vi "Init Coil Calibration.vi"(0 "Magnet ID":string, 1 "# Power Supplies":u32(slide)=4 min=1 max=4 step=1 scale=1.0..4.0, 3 "error in (no error)":errorcluster) -> (4 "File Name":string, 5 "I Scale Max":dbl, 6 "Magnet Configuration Data":T1 {"Scale Factors" format="%.3f"; "Offsets" format="%.3f"; "Temp Coef" format="%.4g"; "Maximum Coil Currents" format="%.2g"; "Coil Inductances" format="%.3g"; "Pressure Range" format="%.2f"}, 7 "P Scale Max":dbl, 8 "P Scale Min":dbl, 9 "error out":errorcluster)   [LabVIEW 2018]
doc: "Reads configuration file for the selected magnet from the folder \"Magnet Calibrations\" on the system disk. All comments (lines starting with a '#') are stripped out and the configuration parameters are parsed and output.\nScott Hannahs, NHMFL-FSU, April 1995\nAuthor: Scott Hannahs <sth@magnet.fsu.edu>\nCopyright 2018 Florida State University, All rights reserved."
uses:
  PS Control/Sub Controls/RMPS Magnet Config.ctl
  RMPS Globals.vi
panel:
  # "Tin"
  # "Tout"
  # "Pin"
  # "Pout"
  # "I"
  # "WDTin"
  # "PSEnb"
  # "CellFLT"
  # "WDTout"
  # "BTFlt"
  # "BTvolt"
  # "Va"
  # "Vb"
  # "Vc"
  # "Vd"
  # "Tin"
  # "Tout"
  # "Pin"
  # "Pout"
  # "I"
  # "WDTin"
  # "PSEnb"
  # "CellFLT"
  # "WDTout"
  # "BTFlt"
  # "BTvolt"
  # "Va"
  # "Vb"
  # "Vc"
  # "Vd"
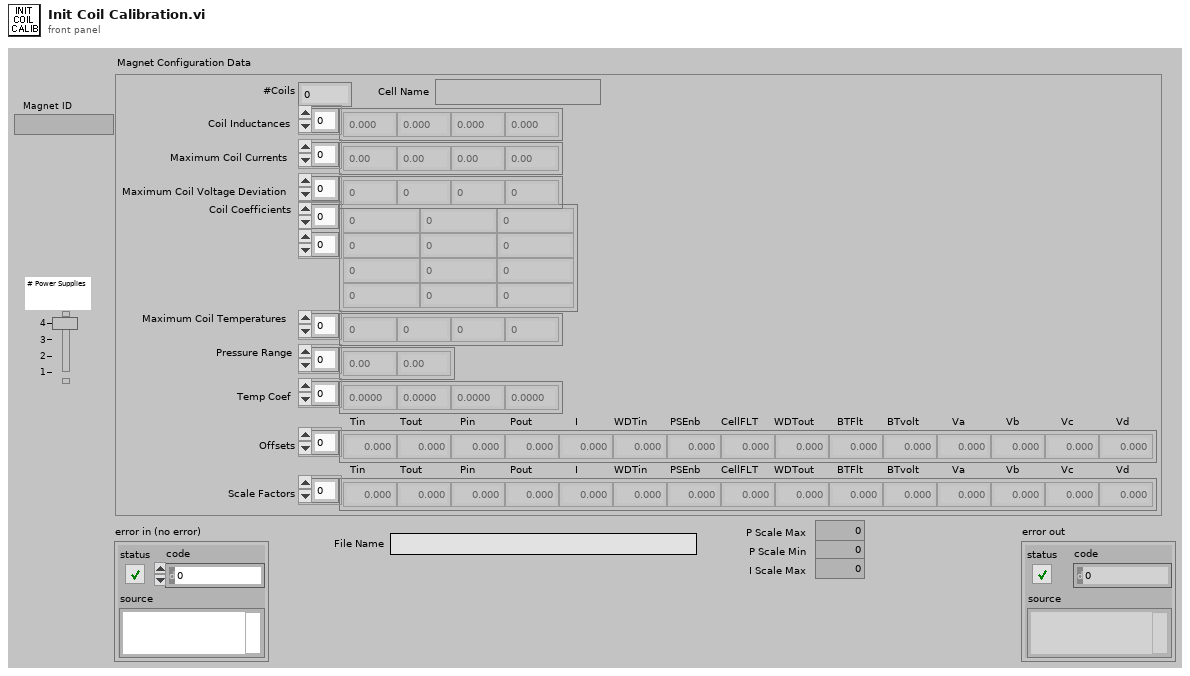
[diagram p1: front panel]
types:
  T1 = typedef "RMPS Magnet Config.ctl" = cluster{"#Coils":u32, "Coil Inductances":dbl[], "Maximum Coil Currents":dbl[], "Maximum Coil Voltage Deviation":dbl[], "Coil Coefficients":dbl[][], "Maximum Coil Temperatures":dbl[], " Pressure Range":dbl[], "Temp Coef":dbl[], "Offsets":dbl[], "Scale Factors":dbl[], "Cell Name":string}
  T2 = cluster{u32, sgl[], sgl[], sgl[], sgl[][], sgl[], sgl[], sgl[], sgl[], sgl[], "Magnet ID":string}
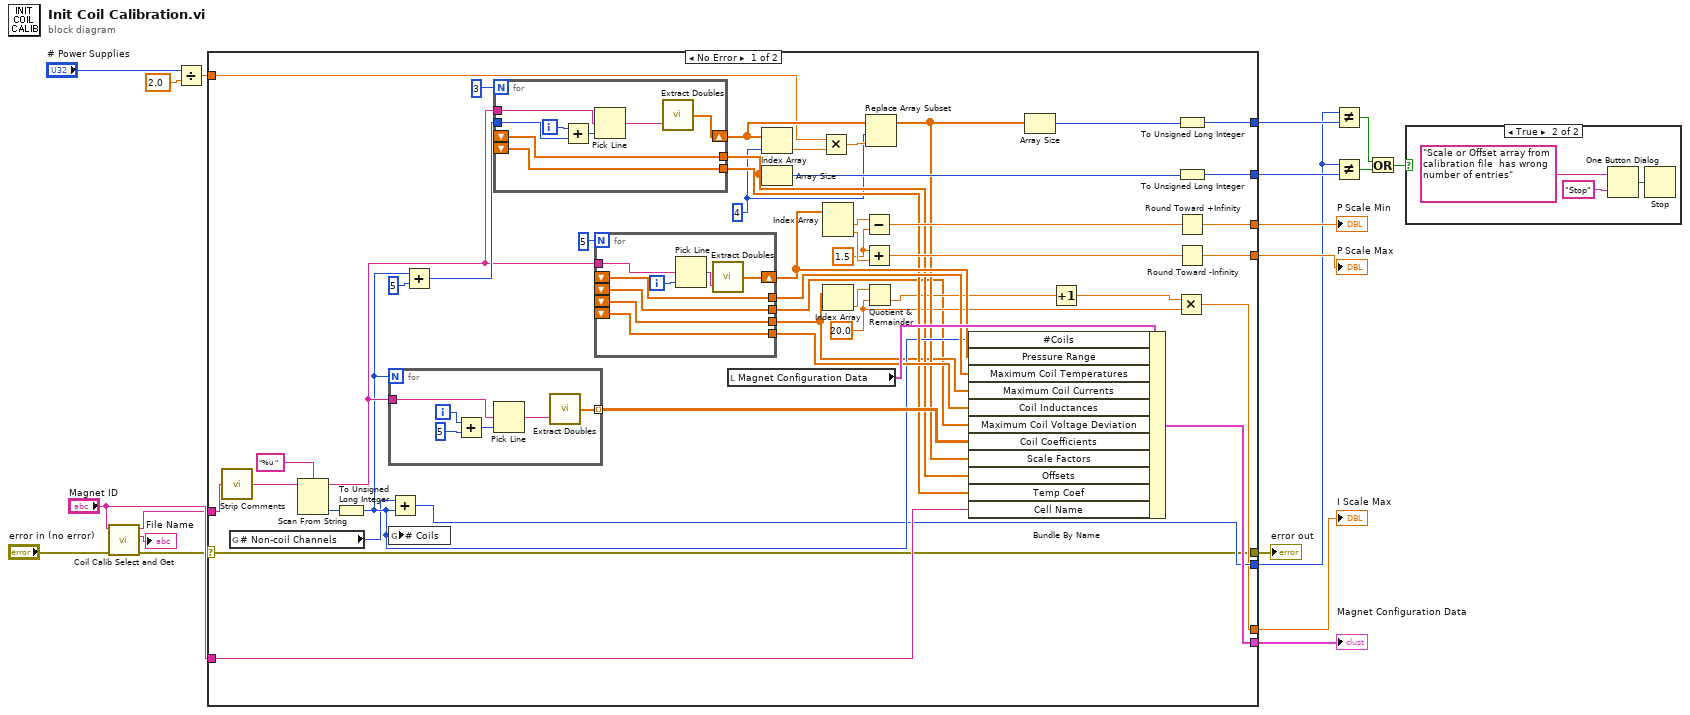
[diagram p0: block diagram]
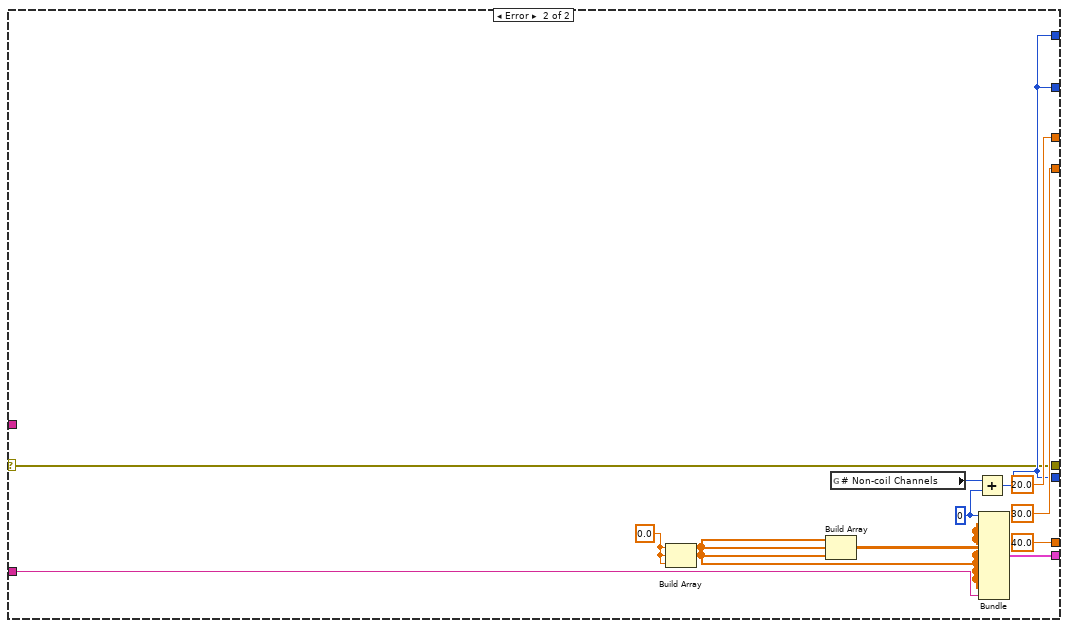
[diagram p3: hidden frame]
diagram:
  n1 = call "Coil Calib Select and Get.vi"("error in (no error)"="error in (no error)", "Magnet ID"="Magnet ID") -> ("error out"=w13:errorcluster, "File Name"=→"File Name":string, "String"=w14:string)  [unwired: 3 in]
  n2 = Divide(x="# Power Supplies", y=sgl 2.0) -> (x/y=w15:sgl)
  n3 = case shown="No Error" w13 {
    selector: w13 -> [w20 w88]
    tunnel: "Magnet ID" -> [w50 w99]
    tunnel: [w48 w96] -> w19
    tunnel: w14 -> [w57 _]
    tunnel: w15 -> [w58 _]
    tunnel: [w40 20.0] -> w12
    tunnel: [w39 30.0] -> w11
    tunnel: [w31 w89] -> w9
    tunnel: [w32 w89] -> w10
    tunnel: [w34 w89] -> w8
    tunnel: [w23 40.0] -> w4
    tunnel: [w20 w88] -> w2
    frame No Error {
      w24 = 20.0 ("y")
      w43 = 1.5 ("y")
      w28 = u32 4 ("y")
      n4 = call "Strip Comments.vi"(1:w57) -> (0:w53:string)
      n5 = global read "RMPS Globals.vi" "# Non-coil Channels"() -> (w33:u32)
      n6 = Scan From String(format string="%u ", input string=w53) -> (remaining string=w54:string, output 1=w55:u32)  [unwired: 3 in, 2 out]
      n7 = To Unsigned Long Integer(number=w55) -> (unsigned 32bit integer=w35:u32)
      n8 = for {
        N: w35 -> [_]
        tunnel: w54 -> [w78]
        tunnel: [w77] -> w47 mode=indexing
        i -> [w75]
        n9 = Add(x=w75, y=5) -> (x+y=w76:i32)
        n10 = Pick Line(multi-line string=w78, line index=w76) -> (output string=w79:string)  [unwired: 1 in]
        n11 = call "Extract Doubles.vi"("String"=w79) -> ("Data"=w77:dbl[])  [unwired: 1 in]
      }
      n12 = global write "RMPS Globals.vi" "# Coils"(w35) -> ()
      n13 = Add(x=w33, y=w35) -> (x+y=w34:u32)
      n14 = Add(x=w35, y=u32 5) -> (x+y=w62:u32)
      n15 = for {
        N: 3 -> [_]
        shift-right: [w69] -> w59
        shift-left: _ -> [w71]
        shift-left: _ -> [w70]
        tunnel: [w71] -> w38
        tunnel: [w70] -> w30
        tunnel: w54 -> [w72]
        tunnel: w62 -> [w66]
        i -> [w67]
        n16 = Add(x=w67, y=w66) -> (x+y=w68:u32)
        n17 = Pick Line(multi-line string=w72, line index=w68) -> (output string=w73:string)  [unwired: 1 in]
        n18 = call "Extract Doubles.vi"("String"=w73) -> ("Data"=w69:dbl[])  [unwired: 1 in]
      }
      n19 = for {
        N: 5 -> [_]
        shift-right: [w80] -> w46
        shift-left: _ -> [w82]
        shift-left: _ -> [w84]
        shift-left: _ -> [w83]
        shift-left: _ -> [w81]
        tunnel: [w82] -> w49
        tunnel: [w84] -> w27
        tunnel: [w83] -> w21
        tunnel: [w81] -> w51
        tunnel: w54 -> [w86]
        i -> [w85]
        n20 = Pick Line(multi-line string=w86, line index=w85) -> (output string=w87:string)  [unwired: 1 in]
        n21 = call "Extract Doubles.vi"("String"=w87) -> ("Data"=w80:dbl[])  [unwired: 1 in]
      }
      n22 = local read "Magnet Configuration Data"() -> (w52:T1)
      n23 = Index Array(array=w59, index=w28) -> (element=w61:dbl)
      n24 = Array Size(array=w30) -> (size(s)=w37:i32)
      n25 = Multiply(x=w58, y=w61) -> (x*y=w60:dbl)
      n26 = Index Array(array=w46) -> (element #1=w45:dbl, element #2=w44:dbl)  [unwired: 2 in]
      n27 = Index Array(array=w27) -> (element=w26:dbl)  [unwired: 1 in]
      n28 = Subtract(x=w45, y=w43) -> (x-y=w42:dbl)
      n29 = Add(x=w43, y=w44) -> (x+y=w41:dbl)
      n30 = Quotient & Remainder(x=w26, y=w24) -> (floor(x/y)=w25:dbl)  [unwired: 1 out]
      n31 = Replace Array Subset(array=w59, new element=w60, index=w28) -> (w29:dbl[])
      n32 = Bundle By Name(cluster=w52, "#Coils"=w35, "Pressure Range"=w46, "Maximum Coil Temperatures"=w51, "Maximum Coil Currents"=w27, "Coil Inductances"=w49, "Maximum Coil Voltage Deviation"=w21, "Coil Coefficients"=w47, "Scale Factors"=w29, "Offsets"=w30, "Temp Coef"=w38, "Cell Name"=w50) -> (w48:T1)
      n33 = Array Size(array=w29) -> (size(s)=w36:i32)
      n34 = Increment(x=w25) -> (x+1=w22:dbl)
      n35 = Multiply(x=w22, y=w24) -> (x*y=w23:dbl)
      n36 = To Unsigned Long Integer(number=w36) -> (unsigned 32bit integer=w32:u32)
      n37 = To Unsigned Long Integer(number=w37) -> (unsigned 32bit integer=w31:u32)
      n38 = Round Toward +Infinity(x=w42) -> (ceil(x): smallest int >= x=w40:dbl)
      n39 = Round Toward -Infinity(1:w41) -> (0:w39:dbl)
    }
    frame Error {
      w91 = u32 0
      w98 = sgl 0.0
      n40 = Build Array(w98, w98, w98) -> (w93:sgl[])
      n41 = Build Array(w93, w93, w93) -> (w97:sgl[][])
      n42 = global read "RMPS Globals.vi" "# Non-coil Channels"() -> (w92:u32)
      n43 = Add(x=w92, y=w91) -> (x+y=w89:u32)
      n44 = Bundle(w91, w93, w93, w93, w97, w93, w93, w93, w93, w93, "Magnet ID"=w99) -> (w96:T2)  [unwired: 1 in]
    }
  }
  "Magnet Configuration Data" <- w19
  "P Scale Min" <- w12
  "P Scale Max" <- w11
  "I Scale Max" <- w4
  "error out" <- w2
  n45 = Not Equal?(x=w8, y=w10) -> (x != y?=w7:bool)
  n46 = Not Equal?(x=w8, y=w9) -> (x != y?=w6:bool)
  n47 = Or(x=w7, y=w6) -> (x .or. y?=w5:bool)
  n48 = case shown="True" w5 {
    frame False {
    }
    frame True {
      n49 = One Button Dialog(message="Scale or Offset array from calibration file  has wrong number of entries", button name ("OK")="Stop") -> (true=w102:bool)
      n50 = Stop(stop? (T)=w102) -> ()
    }
  }
